vi "Set RemotePath.vi"(8 "error in (no error)":errorcluster, 10 "RemotePath":string, 11 "FileTransfer in":refnum<class "FileTransfer.lvclass">) -> (0 "error out":errorcluster, 3 "FileTransfer out":refnum<class "FileTransfer.lvclass">)   [LabVIEW 2015, in "WinSCP.lvlib" / "FileTransfer.lvclass"]
uses:
  FileTransfer.lvclass
  FileTransfer.lvclass/FileTransfer.ctl
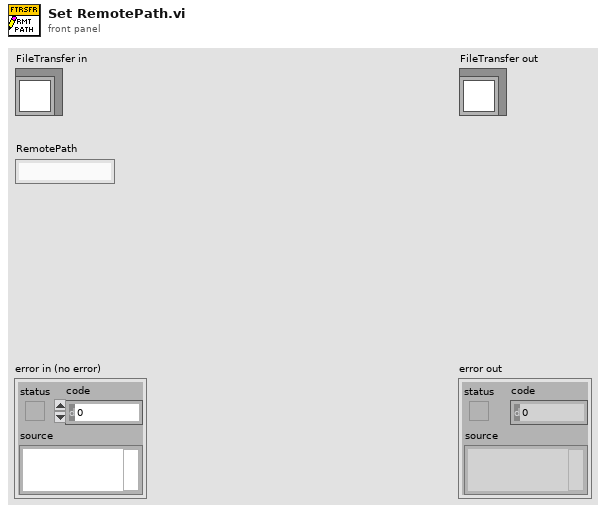
[diagram p1: front panel]
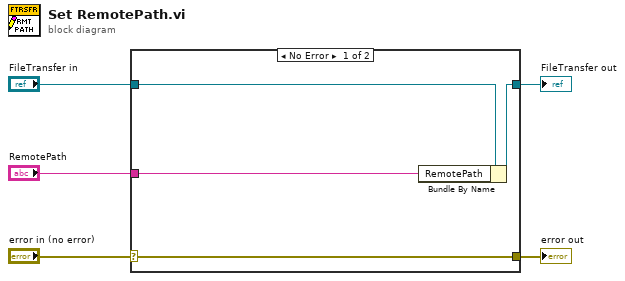
[diagram p0: block diagram]
diagram:
  n1 = case shown="No Error" "error in (no error)" {
    selector: "error in (no error)" -> [w9 w10]
    tunnel: [w9 w10] -> w4
    tunnel: [w7 w11] -> w2
    tunnel: "FileTransfer in" -> [w8 w11]
    tunnel: "RemotePath" -> [w6 _]
    frame No Error {
      n2 = Bundle By Name(cluster=w8, "RemotePath"=w6) -> (w7:refnum<class "FileTransfer.lvclass">)
    }
    frame Error {
    }
  }
  "error out" <- w4
  "FileTransfer out" <- w2
